vi "Read (Single Point).vi"(8 "error in (no error)":errorcluster, 11 "VISA resource name":refnum<visa-resource-name>) -> (0 "error out":errorcluster, 2 "Measurement":dbl, 3 "VISA resource name out":refnum<visa-resource-name>)   [LabVIEW 2020, in "Agilent 34401.lvlib"]
doc: "Reads and returns a single measurement from the instrument."
uses:
  Agilent 34401.lvlib
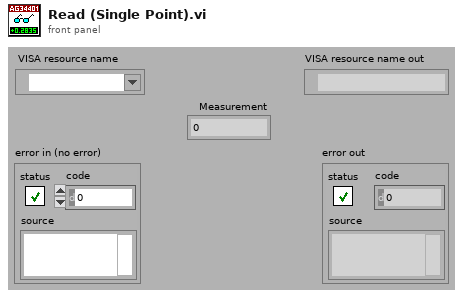
[diagram p1: front panel]
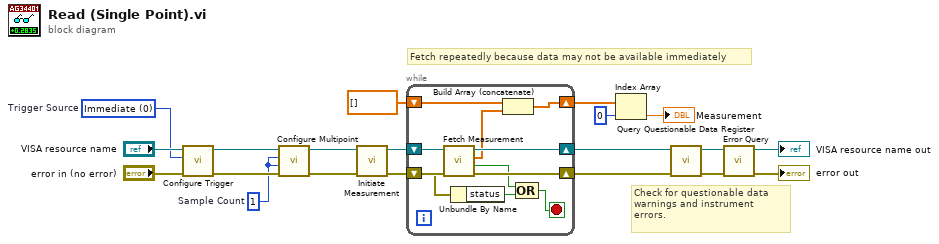
[diagram p0: block diagram]
diagram:
  w7 = u16 0 items=["Immediate", "Software (Bus)", "External", "Internal"]  # Trigger Source
  w6 = 1  # Sample Count
  # "Check for questionable data warnings and instrument errors."
  # "Fetch repeatedly because data may not be available immediately"
  n1 = call "Configure Trigger.vi"("error in (no error)"="error in (no error)", "Trigger Source (0: Immediate)"=w7, "VISA resource name"="VISA resource name") -> ("error out"=w10:errorcluster, "VISA resource name out"=w11:refnum<visa-resource-name>)  [unwired: 7 in]
  n2 = call "Configure Multipoint.vi"("error in (no error)"=w10, "Sample Count (1)"=w6, "Trigger Count (1)"=w6, "VISA resource name"=w11) -> ("error out"=w8:errorcluster, "VISA resource name out"=w9:refnum<visa-resource-name>)  [unwired: 6 in]
  n3 = call "Initiate Measurement.vi"("error in (no error)"=w8, "VISA resource name"=w9) -> ("error out"=w13:errorcluster, "VISA resource name out"=w12:refnum<visa-resource-name>)  [unwired: 8 in]
  n4 = while {
    shift-right: [w30] -> w17
    shift-left: w12 -> [w28]
    shift-right: [w27] -> w16
    shift-left: w13 -> [w29]
    shift-right: [w22] -> w14
    shift-left: dbl[] [] -> [w21]
    stop <- w24 stop-if-true
    n5 = call "Fetch Measurement.vi"("error in (no error)"=w29, "VISA resource name"=w28) -> ("error out"=w27:errorcluster, "End of Data?"=w26:bool, "Measurements"=w23:dbl[], "VISA resource name out"=w30:refnum<visa-resource-name>)  [unwired: 6 in]
    n6 = Unbundle By Name(w27) -> ("status"=w25:bool)
    n7 = Build Array (concatenate)(w21, w23) -> (w22:dbl[])
    n8 = Compound Arithmetic op=OR(w26, w25) -> (w24:bool)
  }
  n9 = Index Array(array=w14, index=0) -> (element=→"Measurement":dbl)
  n10 = call "Query Questionable Data Register.vi"("error in (no error)"=w16, "VISA resource name"=w17) -> ("error out"=w4:errorcluster, "VISA resource name out"=w3:refnum<visa-resource-name>)  [unwired: 7 in, 1 out]
  n11 = call "Error Query.vi"("error in (no error)"=w4, "VISA resource name"=w3) -> ("error out"=→"error out":errorcluster, "VISA resource name out"=→"VISA resource name out":refnum<visa-resource-name>)  [unwired: 6 in, 2 out]
